vi "Self Test.vi"(8 "error in":errorcluster, 11 "ProXR_IO in":refnum<class "ProXR.lvclass">) -> (0 "error out":errorcluster, 3 "ProXR_IO out":refnum<class "ProXR.lvclass">)   [LabVIEW 2019, in "ProXR.lvlib" / "ProXR.lvclass"]
uses:
  Library/ProXR.lvclass
  builds/Instruments/DIG_IO.lvlibp/Library/DIG_IO.lvclass
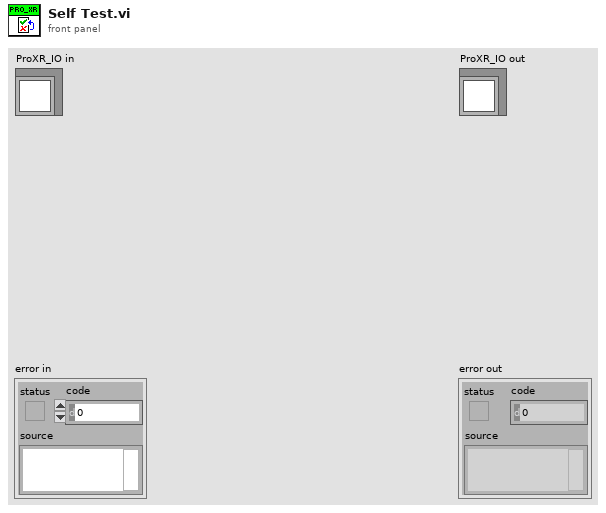
[diagram p1: front panel]
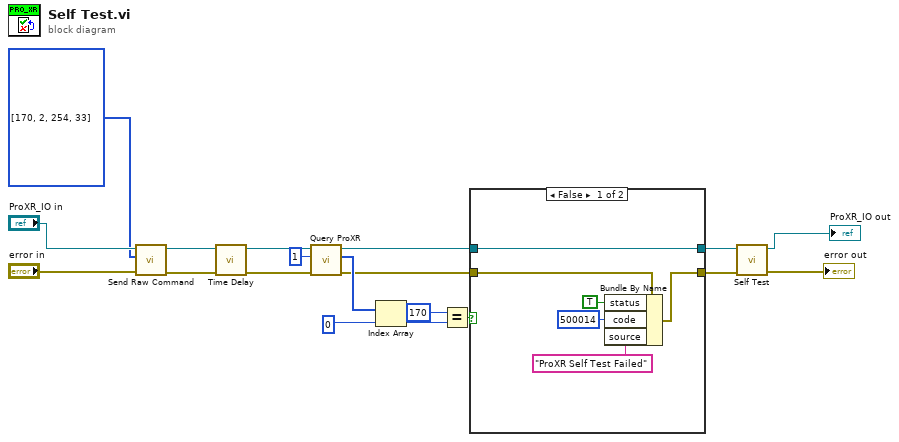
[diagram p0: block diagram]
diagram:
  n1 = call "Send Raw Command.vi"("error in"="error in", "Raw Command"=u8[] [170, 2, 254, 33], "ProXR_IO in"="ProXR_IO in") -> ("error out"=w16:errorcluster, "ProXR_IO out"=w15:refnum<class "ProXR.lvclass">)  [unwired: 7 in]
  n2 = call "Time Delay"("error in (no error)"=w16) -> ("error out"=w1:errorcluster)  [unwired: 10 in]
  n3 = call "Query ProXR.vi"("error in"=w1, "Bytes to Read"=u32 1, "ProXR_IO in"=w15) -> ("error out"=w4:errorcluster, "Response"=w12:u8[], "ProXR_IO out"=w6:refnum<class "ProXR.lvclass">)  [unwired: 6 in]
  n4 = Index Array(array=w12, index=0) -> (element=w10:u8)
  n5 = Equal?(x=u8 170, y=w10) -> (x = y?=w2:bool)
  n6 = case shown="False" w2 {
    tunnel: w6 -> [w24 w26]
    tunnel: [w24 w26] -> w5
    tunnel: w4 -> [w23 w25]
    tunnel: [w21 w25] -> w3
    frame False {
      n7 = Bundle By Name(cluster=w23, "status"=TRUE, "code"=500014, "source"="ProXR Self Test Failed") -> (w21:errorcluster)
    }
    frame True {
    }
  }
  n8 = call-parent "Self Test.vi"("error in"=w3, "Instruments in"=w5) -> ("error out"=→"error out":errorcluster, "Instruments out"=→"ProXR_IO out":refnum<class "ProXR.lvclass">)  [unwired: 8 in]
